vi "读取波形文件.vi"() -> ()   [LabVIEW 2010]
panel:
  in  "起始记录号":i32
  in  "停止":bool
  out "采样间隔":dbl format="%.4f"
  in  "文件路径及名称":path=path "F:/bookoflv7/10.21/c11/PRO10/wf1"
  out "波形图":waveform(dbl)[](graph)
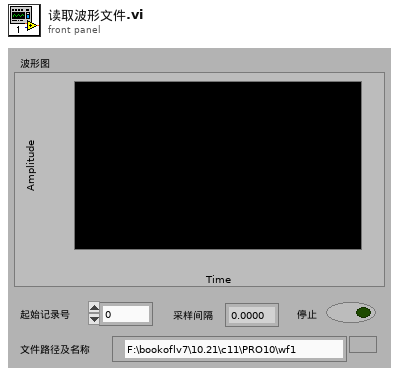
[diagram p1: front panel]
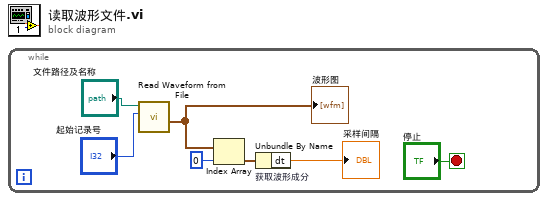
[diagram p0: block diagram]
diagram:
  n1 = while {
    stop <- "停止" stop-if-true
    n2 = call <vilib>:"Read Waveform from File.vi"("offset (records:0)"="起始记录号", "file path (dialog if empty)"="文件路径及名称") -> ("all waveforms in record"=w1:waveform(dbl)[])  [unwired: 4 in, 3 out]
    "波形图" <- w1
    n3 = Index Array(array=w1, index=0) -> (element=w4:waveform(dbl))
    n4 = Unbundle By Name "获取波形成分"(w4) -> ("dt"=→"采样间隔":dbl)
  }
